vi "debug print front panel.vi"(11 "Device Info":T1 {"Outputs"."Output Data References"."Holding Registers" format="%.0x"; "Outputs"."Output Data References"."Coils" format="%.0x"; "Outputs"."Output References"."Holding Registers" format="%.0x"; "Outputs"."Output References"."Coils" format="%.0x"; "Inputs"."Input Data References"."Input Registers" format="%.0x"; "Inputs"."Input Data References"."Discrete Inputs" format="%.0x"; "Inputs"."Input References"."Input Registers" format="%.0x"; "Inputs"."Input References"."Discrete Inputs" format="%.0x"; "Interface Data"."Serial Settings"."parity (even)" items=["None", "Odd", "Even", "Mark", "Space"]; "Interface Data"."Serial Settings"."flow control (none)" items=["None", "XON/XOFF", "RTS/CTS", "XON/XOFF & RTS/CTS", "DTR/DSR", "XON/XOFF & DTR/DSR"]}) -> ()   [LabVIEW 2015]
uses:
  Shared/Device Info.ctl
  Shared/Controls/Interface Type.ctl
  Shared/Controls/Data Model/TCP Settings.ctl
  Shared/Controls/Data Model/Serial Settings.ctl
  Shared/Controls/Data Model/Inputs.ctl
  Shared/Controls/Data Model/Input Channel Data.ctl
  Shared/Controls/Data Model/Channel.ctl
  Modbus Type.ctl
  Shared/Controls/Data Model/Input References.ctl
  <vilib>/NI Veristand/Custom Device API/Custom Device Item Ref.ctl
  Shared/Controls/Data Model/Input Data References.ctl
  <vilib>/NI Veristand/Custom Device API/Data Reference.ctl
  Shared/Controls/Data Model/Input Data.ctl
  Shared/Controls/Data Model/Outputs.ctl
  Shared/Controls/Data Model/Output Channel Data.ctl
  Shared/Controls/Data Model/Output References.ctl
  Shared/Controls/Data Model/Output Data References.ctl
  Shared/Controls/Data Model/Output Data.ctl
  Modbus Master System Explorer.lvlib
  Shared/Modbus Master Shared.lvlib
  <vilib>/NI Veristand/Custom Device API/Custom Device API.lvlib
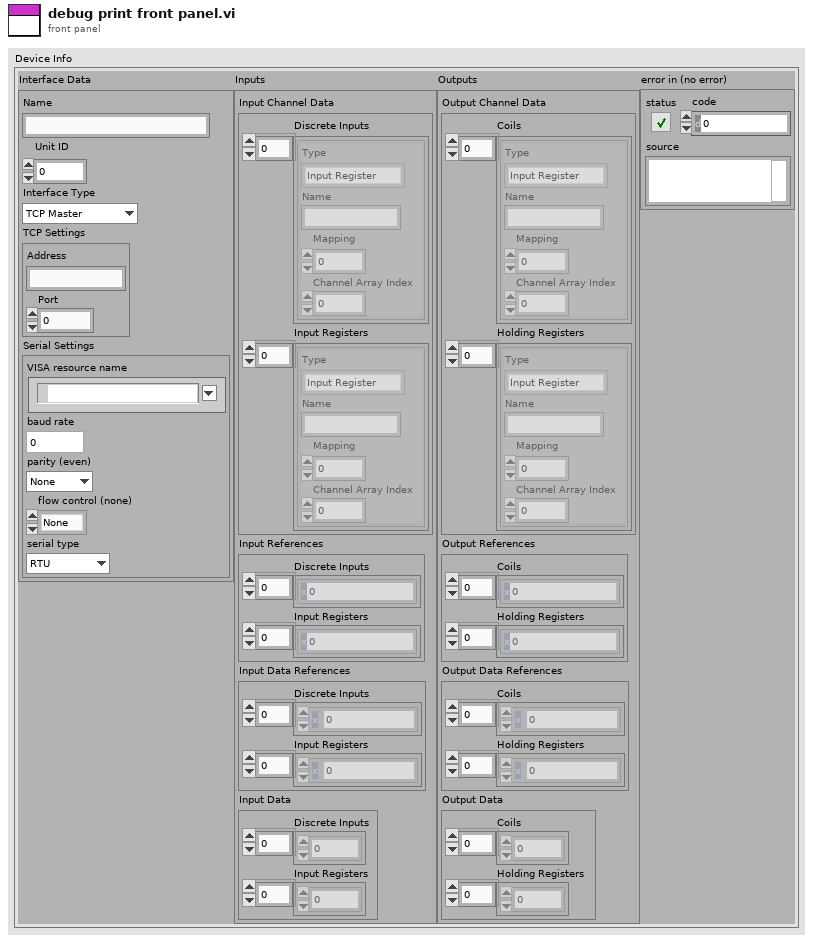
[diagram p1: front panel]
types:
  T1 = typedef "Modbus Master Shared.lvlib/Device Info.ctl" = cluster{"Interface Data":cluster{"Name":string, "Unit ID":u8, "Interface Type":T2, "TCP Settings":T3, "Serial Settings":T4}, "Inputs":T5, "Outputs":T14, "error in (no error)":errorcluster}
  T2 = typedef "Modbus Master System Explorer.lvlib/Interface Type.ctl" = enum16{"TCP Master", "Serial Master"}
  T3 = typedef "Modbus Master Shared.lvlib/TCP Settings.ctl" = cluster{"Address":string, "Port":u16}
  T4 = typedef "Modbus Master Shared.lvlib/Serial Settings.ctl" = cluster{"VISA resource name":refnum<visa-resource-name>, "baud rate":u32, "parity (even)":u16, "flow control (none)":u16, "serial type":enum16{"RTU", "ASCII"}}
  T5 = typedef "Modbus Master Shared.lvlib/Inputs.ctl" = cluster{"Input Channel Data":T6, "Input References":T9, "Input Data References":T11, "Input Data":T13}
  T6 = typedef "Modbus Master Shared.lvlib/Input Channel Data.ctl" = cluster{"Discrete Inputs":T7[], "Input Registers":T7[]}
  T7 = typedef "Modbus Master Shared.lvlib/Channel.ctl" = cluster{"Type":T8, "Name":string, "Mapping":u16, "Channel Array Index":i32}
  T8 = typedef "Modbus Master Shared.lvlib/Modbus Type.ctl" = enum16{"Coil", "Discrete Input", "Holding Register", "Input Register"}
  T9 = typedef "Modbus Master Shared.lvlib/Input References.ctl" = cluster{"Discrete Inputs":T10[], "Input Registers":T10[]}
  T10 = typedef "Custom Device API.lvlib/Custom Device Item Ref.ctl" = u64
  T11 = typedef "Modbus Master Shared.lvlib/Input Data References.ctl" = cluster{"Discrete Inputs":T12[], "Input Registers":T12[]}
  T12 = typedef "Custom Device API.lvlib/Data Reference.ctl" = i32
  T13 = typedef "Modbus Master Shared.lvlib/Input Data.ctl" = cluster{"Discrete Inputs":dbl[], "Input Registers":dbl[]}
  T14 = typedef "Modbus Master Shared.lvlib/Outputs.ctl" = cluster{"Output Channel Data":T15, "Output References":T16, "Output Data References":T17, "Output Data":T18}
  T15 = typedef "Modbus Master Shared.lvlib/Output Channel Data.ctl" = cluster{"Coils":T7[], "Holding Registers":T7[]}
  T16 = typedef "Modbus Master Shared.lvlib/Output References.ctl" = cluster{"Coils":T10[], "Holding Registers":T10[]}
  T17 = typedef "Modbus Master Shared.lvlib/Output Data References.ctl" = cluster{"Coils":T12[], "Holding Registers":T12[]}
  T18 = typedef "Modbus Master Shared.lvlib/Output Data.ctl" = cluster{"Coils":dbl[], "Holding Registers":dbl[]}
  T19 = typedef "imagedata.ctl" = cluster{"image type":i32, "image depth":i32, "image":u8[], "mask":u8[], "colors":u32[], "Rectangle":cluster{"left":i16, "top":i16, "right":i16, "bottom":i16}}
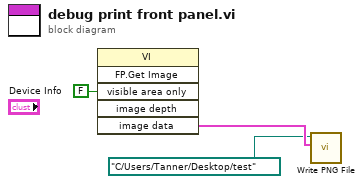
[diagram p0: block diagram]
diagram:
  n1 = invoke class="VI" method="FP.Get Image"("visible area only"=FALSE ("Visible Area Only")) -> ("image data"=w3:T19)  [unwired: 5 in, 5 out]
  n2 = call <vilib>:"Write PNG File.vi"("image data"=w3, "path to PNG file"=path "C:/Users/Tanner/Desktop/test") -> ()  [unwired: 8 in, 2 out]
